vi "Timer.vi"(8 "Stop?":bool, 9 "Reset":bool, 10 "Start":bool, 11 "Time (ms)":dbl) -> (1 "Elapsed Time (ms)":dbl, 2 "Counting Down?":bool, 3 "Time Expired?":bool)   [LabVIEW 2017]
uses:
  <userlib>/836-Library/Logic/Logic_Support/TimerStates.ctl
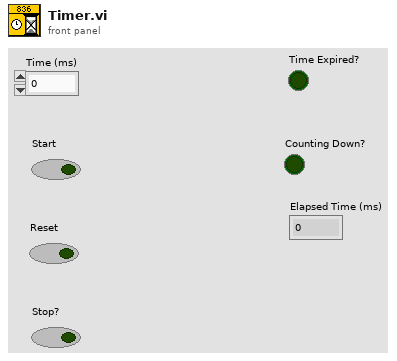
[diagram p1: front panel]
types:
  T1 = typedef "TimerStates.ctl" = enum16{"Idle", "Counting"}
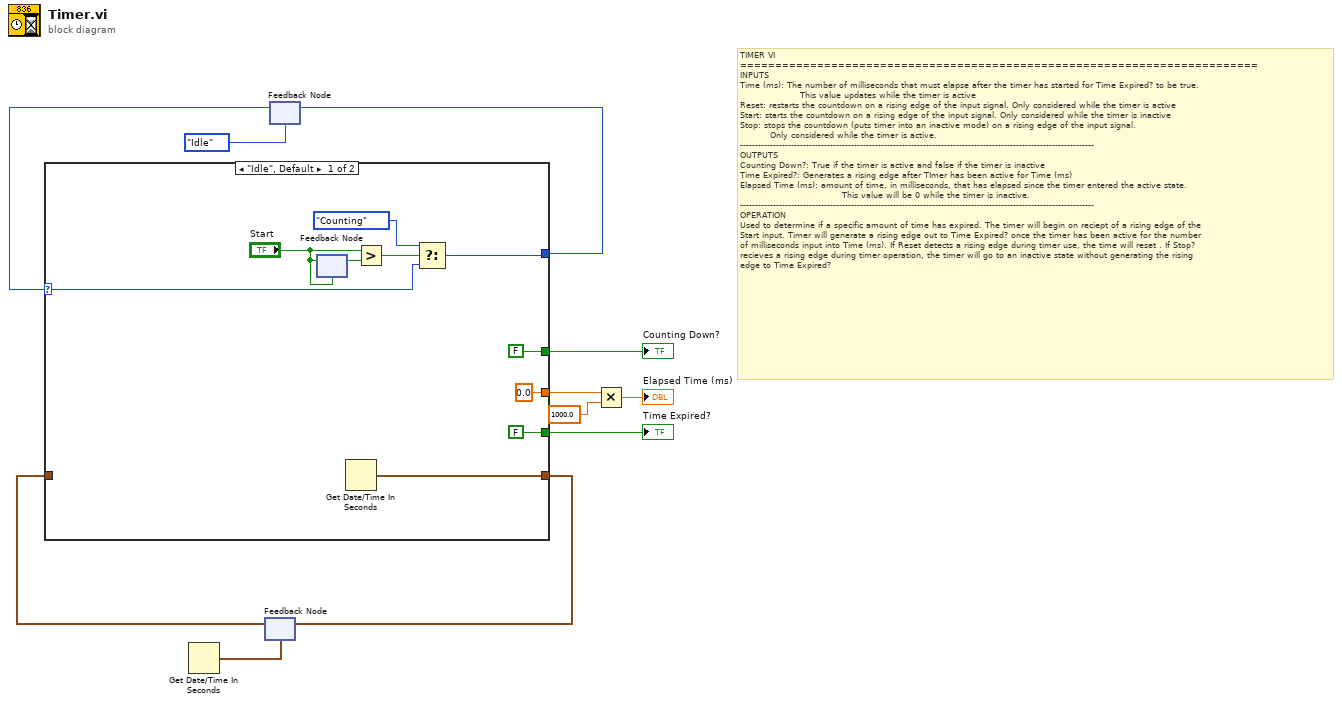
[diagram p0: block diagram]
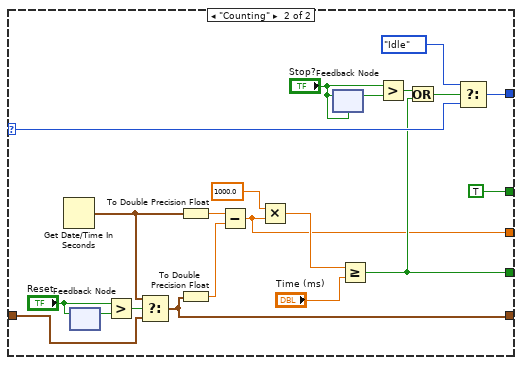
[diagram p2: hidden frame]
diagram:
  # "TIMER VI\n==========================================================================\nINPUTS\nTime (ms): The number of milliseconds that must elapse after the timer has started for Time Expired? to be true. \n                    This value updates while the timer is active\nReset: restarts the countdown on a rising edge of the input signal. Only considered while the timer is active\nStart: starts the countdown on a rising edge of the input signal. Only considered while the timer is inactive \nStop: stops the countdown (puts timer into an inactive mode) on a rising edge of the input signal. \n          Only considered while the timer is active.\n----------------------------------------------------------------------------------------------------------------------\nOUTPUTS\nCounting Down?: True if the timer is active and false if the timer is inactive\nTime Expired?: Generates a rising edge after TImer has been active for Time (ms)\nElapsed Time (ms): amount of time, in milliseconds, that has elapsed since the timer entered the active state. \n                                  This value will be 0 while the timer is inactive.\n----------------------------------------------------------------------------------------------------------------------\nOPERATION\nUsed to determine if a specific amount of time has expired. The timer will begin on reciept of a rising edge of the\nStart input. Timer will generate a rising edge out to Time Expired? once the timer has been active for the number\nof milliseconds input into Time (ms). If Reset detects a rising edge during timer use, the time will reset . If Stop?\nrecieves a rising edge during timer operation, the timer will go to an inactive state without generating the rising\nedge to Time Expired?"
  n1 = Get Date/Time In Seconds() -> (seconds since 1Jan1904=w5:timestamp)
  n2 = feedback #1(w5) -> (w6:timestamp)
  n3 = feedback #2(TimerStates."Idle") -> (w10:T1)
  n4 = case shown="\"Idle\", Default" w10 {
    selector: w10 -> [w19 w32]
    tunnel: [w17 w30] -> w9
    tunnel: [FALSE w28] -> w8
    tunnel: [w15 w34] -> w7
    tunnel: w6 -> [_ w38]
    tunnel: [FALSE TRUE] -> w4
    tunnel: [0.0 w22] -> w3
    frame "Idle", Default {
      n5 = feedback-in #3("Start") -> ()
      n6 = feedback #3("Start") -> (w21:bool)
      n7 = Get Date/Time In Seconds() -> (seconds since 1Jan1904=w15:timestamp)
      n8 = Greater?(x="Start", y=w21) -> (0:w20:bool)
      n9 = Select(t=TimerStates."Counting", s=w20, f=w19) -> (s? t:f=w17:T1)
    }
    frame "Counting" {
      n10 = Get Date/Time In Seconds() -> (seconds since 1Jan1904=w37:timestamp)
      n11 = feedback-in #4("Reset") -> ()
      n12 = feedback #4() -> (w40:bool)  [unwired: 1 in]
      n13 = Greater?(x="Reset", y=w40) -> (0:w39:bool)
      n14 = Select(t=w37, s=w39, f=w38) -> (s? t:f=w34:timestamp)
      n15 = To Double Precision Float(number=w37) -> (double precision float=w36:dbl)
      n16 = To Double Precision Float(number=w34) -> (double precision float=w35:dbl)
      n17 = Subtract(x=w36, y=w35) -> (x-y=w22:dbl)
      n18 = Multiply(x=1000.0, y=w22) -> (x*y=w24:dbl)
      n19 = feedback-in #5("Stop?") -> ()
      n20 = feedback #5("Stop?") -> (w27:bool)
      n21 = Greater Or Equal?(x=w24, y="Time (ms)") -> (x >= y?=w28:bool)
      n22 = Greater?(x="Stop?", y=w27) -> (0:w25:bool)
      n23 = Or(x=w25, y=w28) -> (x .or. y?=w29:bool)
      n24 = Select(t=TimerStates."Idle", s=w29, f=w32) -> (s? t:f=w30:T1)
    }
  }
  "Time Expired?" <- w8
  "Counting Down?" <- w4
  n25 = feedback-in #1(w7) -> ()
  n26 = feedback-in #2(w9) -> ()
  n27 = Multiply(x=w3, y=1000.0) -> (x*y=→"Elapsed Time (ms)":dbl)
